vi "AuthEncryptionKeyResponse_Create.vi"(7 "Header":T3, 8 "error in (no error)":errorcluster, 9 "ResponseError":errorcluster, 10 "AuthEncryptionKeyResponse":T1, 11 "IRoutingSource":T2) -> (0 "error out":errorcluster, 3 "Message":T5)   [LabVIEW 2017]
uses:
  <vilib>/addons/InsightCM/MessageBus/Base/controls/Message.ctl
  <vilib>/addons/InsightCM/MessageBus/Base/controls/MessageHeader.ctl
  <vilib>/addons/InsightCM/MessageBus/Base/controls/KeyValuePair.ctl
  <vilib>/addons/InsightCM/MessageBus/Base/controls/IRoutingSource.ctl
  <vilib>/addons/InsightCM/MessageBus/MessageLibrary/Authentication/controls/AuthEncryptionKeyResponseBody.ctl
  <vilib>/addons/InsightCM/MessageBus/Base/controls/MessageClassType.ctl
  <vilib>/addons/InsightCM/Utilities/PropertyHelpers/PropertyHelpers.lvlib
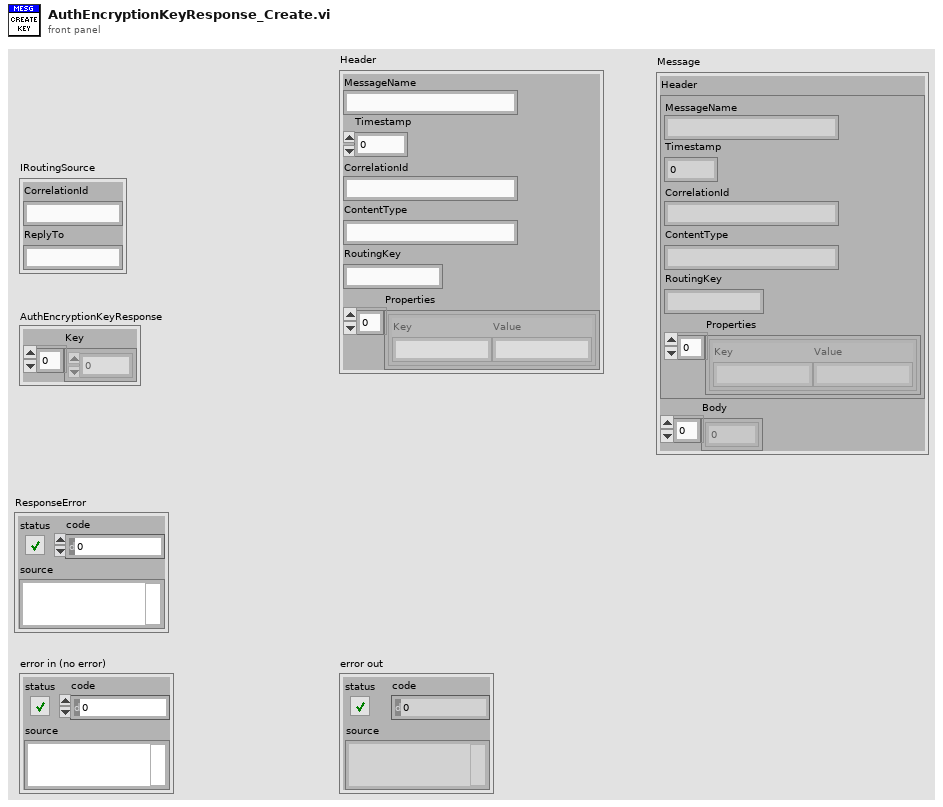
[diagram p1: front panel]
types:
  T1 = typedef "AuthEncryptionKeyResponseBody.ctl" = cluster{"Key":u8[]}
  T2 = typedef "IRoutingSource.ctl" = cluster{"CorrelationId":string, "ReplyTo":string}
  T3 = typedef "MessageHeader.ctl" = cluster{"MessageName":string, "Timestamp":i64, "CorrelationId":string, "ContentType":string, "RoutingKey":string, "Properties":T4[]}
  T4 = typedef "KeyValuePair.ctl" = cluster{"Key":string, "Value":string}
  T5 = typedef "Message.ctl" = cluster{"Header":T3, "Body":u8[]}
  T6 = typedef "MessageClassType.ctl" = enum16{"Request", "Response", "Broadcast", "RoutedMessage"}
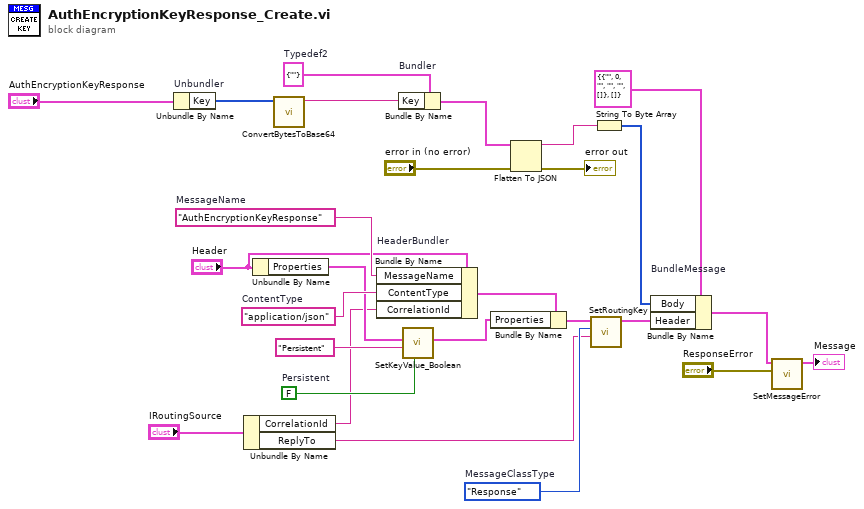
[diagram p0: block diagram]
diagram:
  w3 = cluster{"Key":string} {"Key"=""}  # Typedef2
  w23 = MessageClassType."Response"  # MessageClassType
  w18 = FALSE  # Persistent
  w24 = "AuthEncryptionKeyResponse"  # MessageName
  w21 = "application/json"  # ContentType
  n1 = Unbundle By Name "Unbundler"("AuthEncryptionKeyResponse") -> ("Key"=w2:u8[])
  n2 = Unbundle By Name("IRoutingSource") -> ("CorrelationId"=w8:string, "ReplyTo"=w7:string)
  n3 = Unbundle By Name("Header") -> ("Properties"=w20:T4[])
  n4 = call <vilib>:"ConvertBytesToBase64.vi"("U8 array"=w2) -> ("base64 encoded"=w1:string)  [unwired: 10 in]
  n5 = Bundle By Name "HeaderBundler"(cluster="Header", "MessageName"=w24, "ContentType"=w21, "CorrelationId"=w8) -> (w15:T3)
  n6 = Bundle By Name "Bundler"(cluster=w3, "Key"=w1) -> (w4:cluster{"Key":string})
  n7 = call <vilib>:"SetKeyValue_Boolean.vi"("value"=w18, "key"="Persistent" ("Key"), "key value pairs"=w20) -> ("key value pairs out"=w14:T4[])  [unwired: 8 in]
  n8 = Bundle By Name(cluster=w15, "Properties"=w14) -> (w16:T3)
  n9 = Flatten To JSON(anything=w4, error in (no error)="error in (no error)") -> (JSON string=w6:string, 11:→"error out":errorcluster)  [unwired: 1 in]
  n10 = call <vilib>:"SetRoutingKey.vi"("SendTo"=w7, "MessageClassType"=w23, "Message Header in"=w16) -> ("Message Header out"=w17:T3)  [unwired: 8 in]
  n11 = String To Byte Array(string=w6) -> (unsigned byte array=w26:u8[])
  n12 = Bundle By Name "BundleMessage"(cluster=T5 {"Header"={"MessageName"="", "Timestamp"=0, "CorrelationId"="", "ContentType"="", "RoutingKey"="", "Properties"=[]}, "Body"=[]} ("Message"), "Body"=w26, "Header"=w17) -> (w12:T5)
  n13 = call <vilib>:"SetMessageError.vi"("error"="ResponseError", "message in"=w12) -> ("message out"=→"Message":T5)  [unwired: 9 in]
